vi "Test_log_temperature_Peregrine.vi"() -> ()   [LabVIEW 2019]
panel:
  out "Temperature sensor":dbl(graph)
  in  "COM Port for serial\nconnection. Check device\nmanager.":string
  out "Decoded value":dbl
  in  "Stop measuring":bool
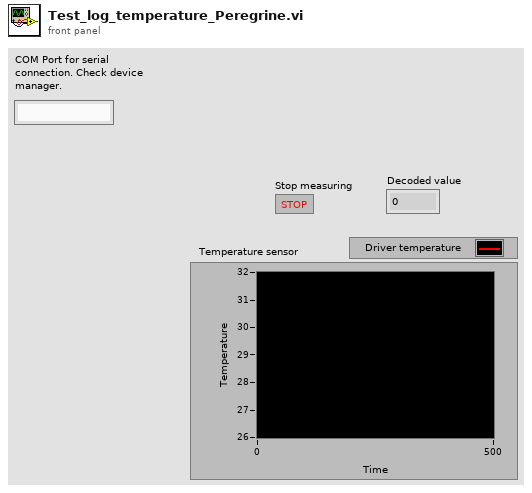
[diagram p1: front panel]
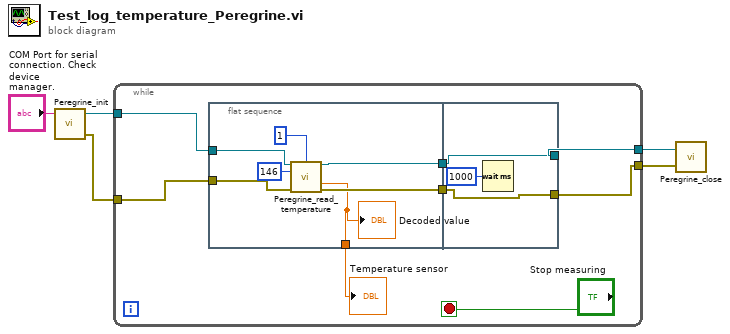
[diagram p0: block diagram]
diagram:
  n1 = call "Peregrine_init.vi"("COM Port for serial\nconnection. Check device\nmanager."="COM Port for serial\nconnection. Check device\nmanager.") -> ("error out"=w3:errorcluster, "Handle out"=w5:refnum<visa-resource-name>)  [unwired: 3 in]
  n2 = while {
    tunnel: w5 -> [w12]
    tunnel: [w10] -> w4
    tunnel: w3 -> [w9]
    tunnel: [w7] -> w2
    stop <- "Stop measuring" stop-if-true
    n3 = flat-sequence {
      tunnel: w12 -> [w20]
      tunnel: [w19] -> w11
      tunnel: w9 -> [w18]
      tunnel: [w17] -> w8
      tunnel: [w14] -> w6
      tunnel: [w22] -> w10
      tunnel: w11 -> [w22]
      tunnel: w8 -> [w21]
      tunnel: [w21] -> w7
      frame #0 {
        n4 = call "Peregrine_read_temperature.vi"("Handle in"=w20, "Address"=u8 1, "i2c address"=u32 146, "error"=w18) -> ("Handle out"=w19:refnum<visa-resource-name>, "Decoded value"=w14:dbl, "error out"=w17:errorcluster)  [unwired: 6 in, 3 out]
        "Decoded value" <- w14
      }
      frame #1 {
        n5 = Wait (ms)(milliseconds to wait=u32 1000) -> ()  [unwired: 1 out]
      }
    }
    "Temperature sensor" <- w6
  }
  n6 = call "Peregrine_close.vi"("error in (no error)"=w2, "Handle in"=w4) -> ()  [unwired: 1 in, 1 out]
